vi "readChar.vi"(9 "Legnth":i32=8, 10 "Offset":i32, 11 "Buffer INÂ":string) -> (1 "Char":string, 2 "Offset+Length":i32, 3 "Buffer OUT":string)   [LabVIEW 2017, in "HEKAdat.lvclass"]
uses:
  HEKAdat.lvclass
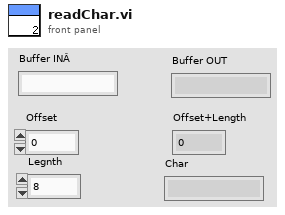
[diagram p1: front panel]
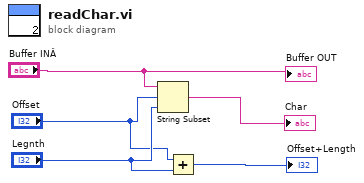
[diagram p0: block diagram]
diagram:
  n1 = String Subset(string="Buffer INÂ", offset (0)="Offset", length (rest)="Legnth") -> (substring=→"Char":string)
  n2 = Add(x="Offset", y="Legnth") -> (x+y=→"Offset+Length":i32)
  "Buffer OUT" <- "Buffer INÂ"
